vi "LoadConfig.vi"(6 "UIMsgReg.":bool, 8 "error in (no error)":errorcluster, 9 "sub-syst Cfg":T1, 10 "UIMsg":refnum<class "SendMessage.lvclass">, 11 "VXMx2 in":refnum<class "VXMx2.lvclass">) -> (0 "error out":errorcluster, 3 "VXMx2 out":refnum<class "VXMx2.lvclass">)   [LabVIEW 2019, in "VXMx2.lvclass"]
doc: "Load properties into the object.\nInit the UI message registered boolean, and handle the case where this is a reload by actually checking the UI Message object."
uses:
  VXMx2.lvclass
  SendMessage/SendMessage.lvclass
  VXMCfg/sub-syst.n.ctl
  VXMx2.lvclass/VXMx2.ctl
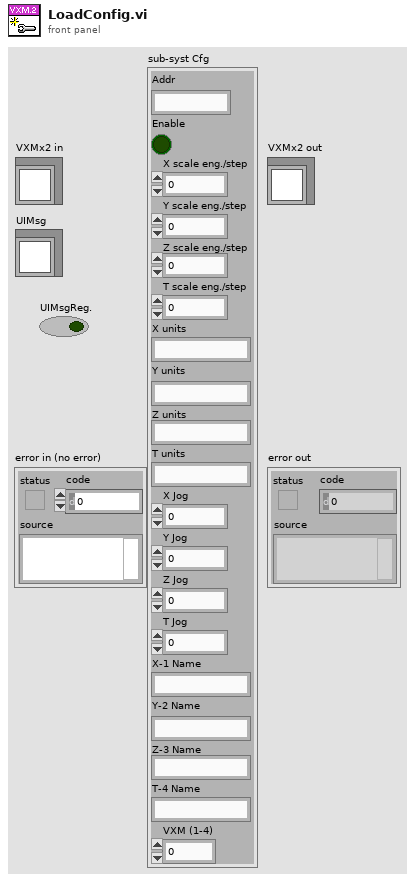
[diagram p1: front panel]
types:
  T1 = typedef "sub-syst.n.ctl" = cluster{"Addr":string, "Enable":bool, "X scale eng./step":dbl, "Y scale eng./step":dbl, "Z scale eng./step":dbl, "T scale eng./step":dbl, "X units":string, "Y units":string, "Z units":string, "T units":string, "X Jog":dbl, "Y Jog":dbl, "Z Jog":dbl, "T Jog":dbl, "X-1 Name":string, "Y-2 Name":string, "Z-3 Name":string, "T-4 Name":string, "VXM (1-4)":i32}
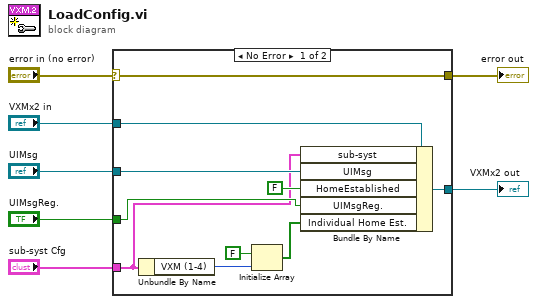
[diagram p0: block diagram]
diagram:
  n1 = case shown="No Error" "error in (no error)" {
    selector: "error in (no error)" -> [w17 w19]
    tunnel: [w17 w19] -> w6
    tunnel: [w16 w18] -> w4
    tunnel: "VXMx2 in" -> [w15 w18]
    tunnel: "UIMsg" -> [w14 _]
    tunnel: "sub-syst Cfg" -> [w11 _]
    tunnel: "UIMsgReg." -> [w12 _]
    frame No Error {
      n2 = Unbundle By Name(w11) -> ("VXM (1-4)"=w10:i32)
      n3 = Initialize Array(FALSE, w10) -> (w8:bool[])
      n4 = Bundle By Name(cluster=w15, "sub-syst"=w11, "UIMsg"=w14, "HomeEstablished"=FALSE ("Homed"), "UIMsgReg."=w12, "Individual Home Est."=w8) -> (w16:refnum<class "VXMx2.lvclass">)
    }
    frame Error {
    }
  }
  "error out" <- w6
  "VXMx2 out" <- w4
